vi "Configure MCCW State.vi"(8 "error in (no error)":errorcluster, 10 "State":bool, 11 "VSG-SMBV in":refnum<class "VSG-SMBV.lvclass">) -> (0 "error out":errorcluster, 3 "VSG-SMBV out":refnum<class "VSG-SMBV.lvclass">)   [LabVIEW 2020, in "VSG-SMBV.lvclass"]
uses:
  VSG-SMBV.lvclass
  C:/Sandbox/Git_Sandbox/WiSpry Test Framework source code (LV20)/WiSpry Test Framework/Instruments/Instrument.lvclass
  Instrument.lvclass/Instrument.ctl
  Instrument.lvclass
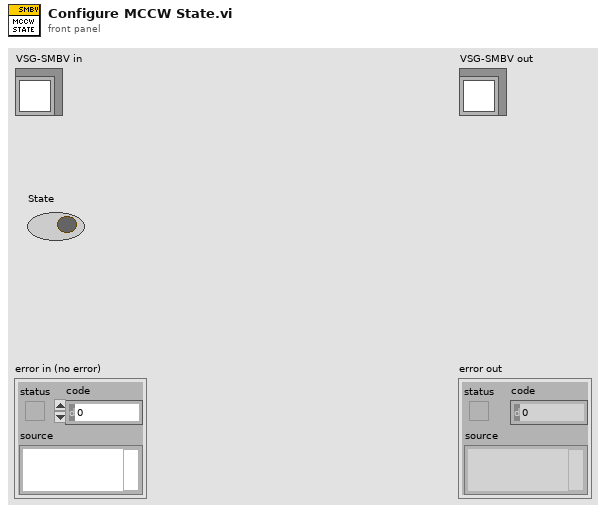
[diagram p1: front panel]
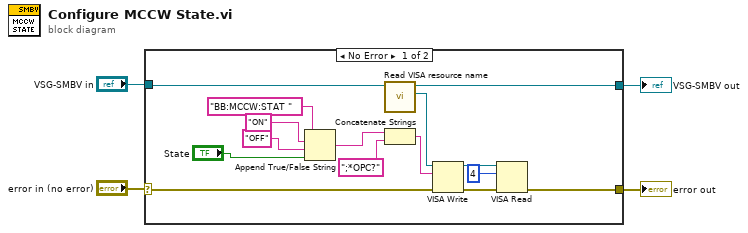
[diagram p0: block diagram]
diagram:
  n1 = case shown="No Error" "error in (no error)" {
    selector: "error in (no error)" -> [w13 w20]
    tunnel: "VSG-SMBV in" -> [w19 w21]
    tunnel: [w9 w21] -> w1
    tunnel: [w5 w20] -> w2
    frame No Error {
      n2 = Append True/False String(1:"State", 2:"OFF" ("false string"), 3:"ON" ("true string"), 4:"BB:MCCW:STAT " ("string (\"\")")) -> (0:w12:string)
      n3 = call "Read VISA resource name.vi"("Instrument in"=w19) -> ("VISA resource name"=w14:refnum<visa-resource-name>, "Instrument out"=w9:refnum<class "VSG-SMBV.lvclass">)  [unwired: 9 in]
      n4 = Concatenate Strings(w12, ";*OPC?" ("string")) -> (w10:string)
      n5 = VISA Write(VISA resource name=w14, write buffer=w10, error in (no error)=w13) -> (VISA resource name out=w7:refnum<visa-resource-name>, error out=w8:errorcluster)  [unwired: 1 out]
      n6 = VISA Read(VISA resource name=w7, byte count=u32 4, error in (no error)=w8) -> (error out=w5:errorcluster)  [unwired: 3 out]
    }
    frame Error {
    }
  }
  "error out" <- w2
  "VSG-SMBV out" <- w1
